vi "Comprar UI.vi"(8 "error in (no error)":errorcluster, 11 "User Interface in":refnum<class "User Interface.lvclass">) -> (0 "error out":errorcluster, 3 "User Interface out":refnum<class "User Interface.lvclass">)   [LabVIEW 2020, in "User Interface.lvlib" / "User Interface.lvclass"]
uses:
  User Interface.lvclass
  User Interface.lvclass/User Interface.ctl
  <vilib>/ActorFramework/Message Enqueuer/Message Enqueuer.lvclass/Message Enqueuer.ctl
  <vilib>/ActorFramework/Message Enqueuer/Enqueue.vi
  Mensajes Messages/Comprar Message Msg/Comprar Message Msg.lvclass
  C:/Program Files (x86)/National Instruments/LabVIEW 2020/vi.lib/ActorFramework/Message/Message.lvclass
  <vilib>/ActorFramework/Message Priority Queue/Priority Enqueue.vi
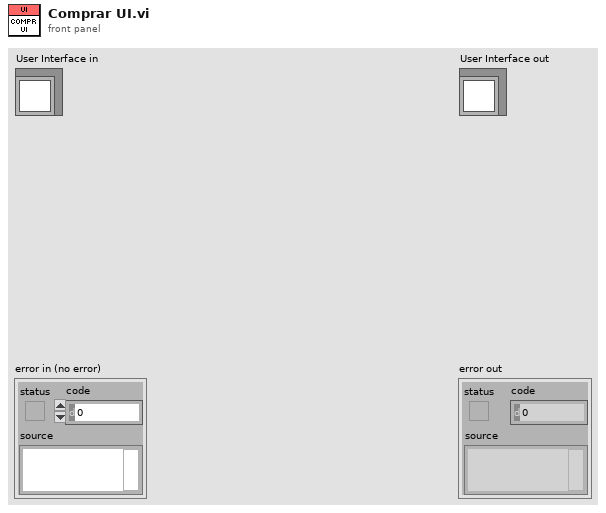
[diagram p1: front panel]
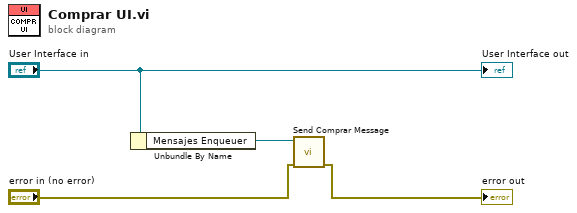
[diagram p0: block diagram]
diagram:
  n1 = Unbundle By Name("User Interface in") -> ("Mensajes Enqueuer"=w3:refnum<class "Message Enqueuer.lvclass">)
  n2 = call "Send Comprar Message.vi"("error in (no error)"="error in (no error)", "Message Enqueuer"=w3) -> ("error out"=→"error out":errorcluster)  [unwired: 8 in, 1 out]
  "User Interface out" <- "User Interface in"
